vi "catch array get.vi"(11 "main-national data":T1) -> (0 "finish?":bool, 3 "main data out":T1)   [LabVIEW 2019]
uses:
  ctl/main data-national.ctl
  ctl/position set.ctl
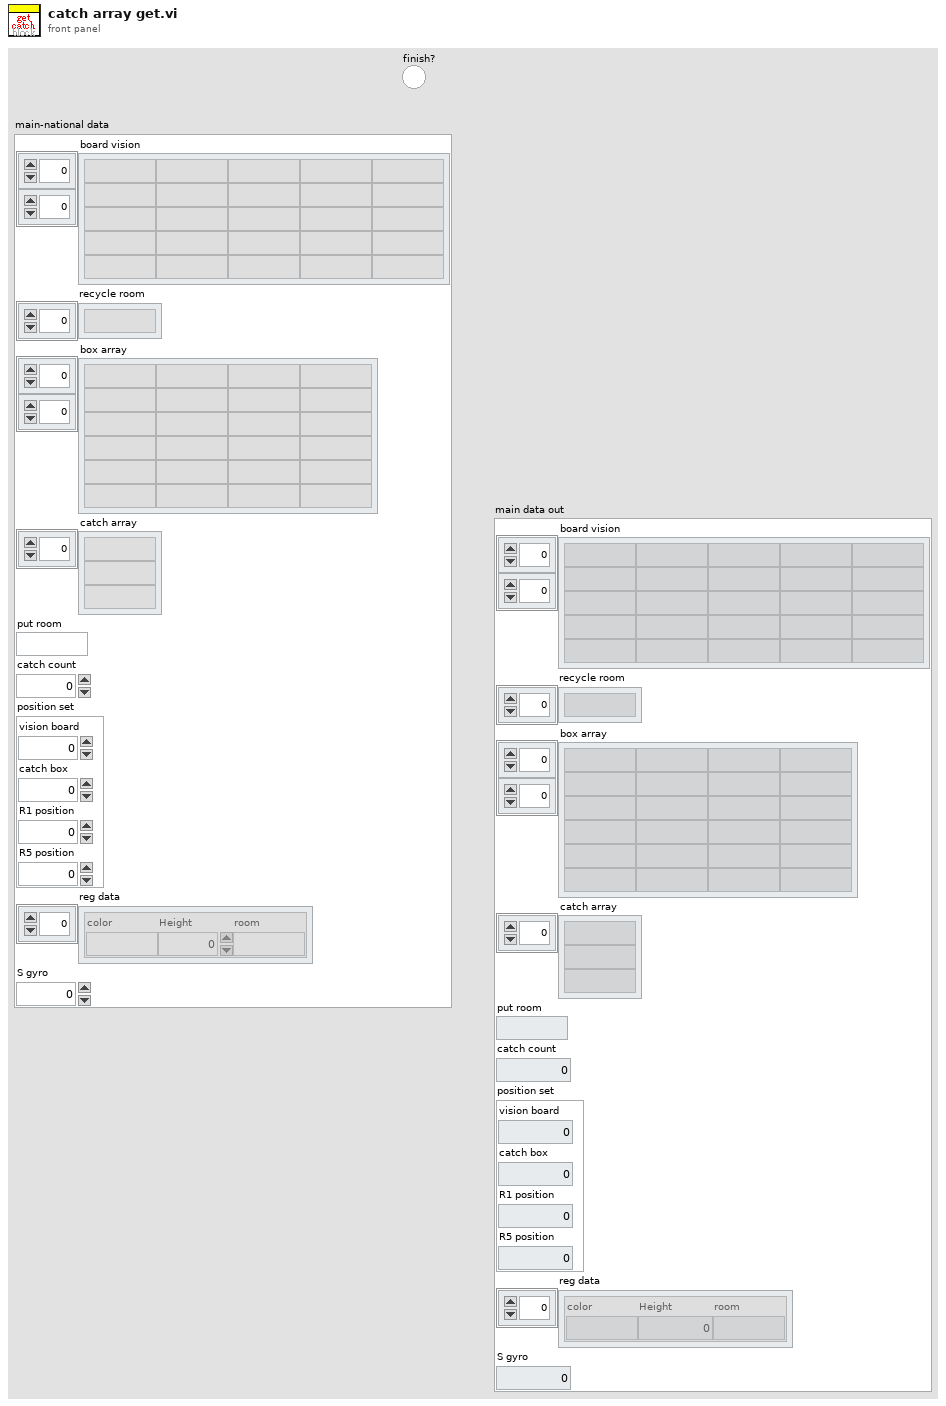
[diagram p1: front panel]
types:
  T1 = typedef "main data-national.ctl" = cluster{"board vision":string[][], "recycle room":string[], "box array":string[][], "catch array":string[], "put room":string, "catch count":dbl, "position set":T2, "reg data":cluster{"color":string, "Height":i32, "room":string}[], "S gyro":dbl}
  T2 = typedef "position set.ctl" = cluster{"vision board":dbl, "catch box":dbl, "R1 position":dbl, "R5 position":dbl}
  T3 = cluster{"color":string, "Height":i32, "room":string}[]
  T4 = cluster{"color":string, "Height":i32, "room":string}
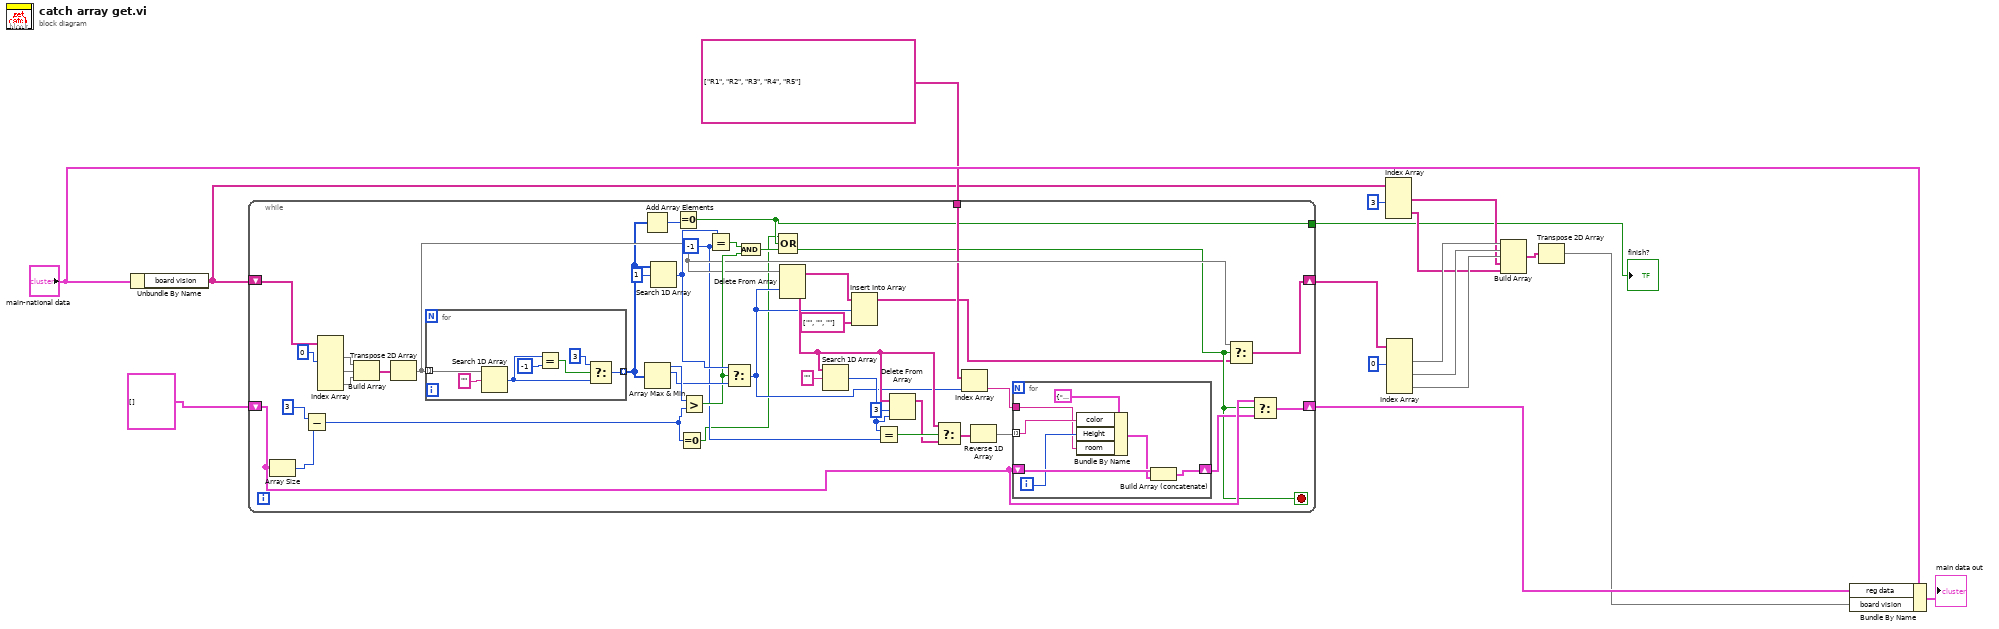
[diagram p0: block diagram]
diagram:
  n1 = Unbundle By Name("main-national data") -> ("board vision"=w10:string[][])
  n2 = while {
    shift-right: [w43] -> w12
    shift-left: w10 -> [w54]
    shift-right: [w31] -> w13
    shift-left: T3 [] ("reg data") -> [w29]
    tunnel: string[] ["R1", "R2", "R3", "R4", "R5"] -> [w33]
    tunnel: [w24] -> w1
    stop <- w25 stop-if-true
    w41 = -1 ("y")
    n3 = Array Size(array=w29) -> (size(s)=w51:i32)
    n4 = Subtract(x=3, y=w51) -> (x-y=w19:i32)
    n5 = Index Array(array=w54, index (col) #1=0 ("disabled index (col)")) -> (element #1=w58:string[], element #2=w56:string[], element #3=w57:string[])  [unwired: 5 in]
    n6 = Build Array(w58, w56, w57) -> (w53:string[][])
    n7 = Transpose 2D Array(2D array=w53) -> (transposed array=w44:string[][])
    n8 = for {
      tunnel: w44 -> [w72] mode=indexing
      tunnel: [w66] -> w27 mode=indexing
      n9 = Search 1D Array(1D array=w72, element="") -> (index of element=w70:i32)  [unwired: 1 in]
      n10 = Equal?(x=w70, y=-1) -> (x = y?=w68:bool)
      n11 = Select(t=3, s=w68, f=w70) -> (s? t:f=w66:i32)
    }
    n12 = Add Array Elements(numeric array=w27) -> (sum=w26:i32)
    n13 = Array Max & Min(array=w27) -> (max value=w50:i32, max index (indices)=w48:i32)  [unwired: 2 out]
    n14 = Search 1D Array(1D array=w27, element=1) -> (index of element=w47:i32)  [unwired: 1 in]
    n15 = Equal To 0?(x=w26) -> (x = 0?=w24:bool)
    n16 = Equal To 0?(x=w19) -> (x = 0?=w18:bool)
    n17 = Greater?(x=w50, y=w19) -> (0:w45:bool)
    n18 = Equal?(x=w47, y=w41) -> (x = y?=w46:bool)
    n19 = Select(t=w47, s=w45, f=w48) -> (s? t:f=w22:i32)
    n20 = And(x=w46, y=w45) -> (x .and. y?=w30:bool)
    n21 = Compound Arithmetic op=OR(w18, w24, w30) -> (w25:bool)
    n22 = Delete From Array(array=w44, index (row)=w22) -> (deleted portion=w39:string[], array with subset deleted=w23:string[][])  [unwired: 2 in]
    n23 = Search 1D Array(1D array=w39, element="") -> (index of element=w37:i32)  [unwired: 1 in]
    n24 = Insert Into Array(array=w23, index (row)=w22, new element=string[] ["", "", ""] ("new element/subarray")) -> (w20:string[][])  [unwired: 1 in]
    n25 = Equal?(x=w37, y=w41) -> (x = y?=w40:bool)
    n26 = Delete From Array(array=w39, length=3, index=w37) -> (array with subset deleted=w36:string[])  [unwired: 1 out]
    n27 = Select(t=w39, s=w40, f=w36) -> (s? t:f=w35:string[])
    n28 = Index Array(array=w33, index=w22) -> (element=w32:string)
    n29 = Reverse 1D Array(array=w35) -> (reversed array=w34:string[])
    n30 = for {
      shift-right: [w64] -> w28
      shift-left: w29 -> [w65]
      tunnel: w34 -> [w62] mode=indexing
      tunnel: w32 -> [w60]
      i -> [w61]
      n31 = Bundle By Name(cluster=T4 {"color"="", "Height"=0, "room"=""} ("Cluster"), "color"=w62, "Height"=w61, "room"=w60) -> (w59:T4)
      n32 = Build Array (concatenate)(w65, w59) -> (w64:T3)
    }
    n33 = Select(t=w44, s=w25, f=w20) -> (s? t:f=w43:string[][])
    n34 = Select(t=w29, s=w25, f=w28) -> (s? t:f=w31:T3)
  }
  "finish?" <- w1
  n35 = Index Array(array=w10, index (col) #1=3 ("disabled index (col)")) -> (element #1=w5:string[], element #2=w4:string[])  [unwired: 3 in]
  n36 = Index Array(array=w12, index (col) #1=0 ("disabled index (col)")) -> (element #1=w8:string[], element #2=w7:string[], element #3=w6:string[])  [unwired: 5 in]
  n37 = Build Array(w8, w7, w6, w5, w4) -> (w3:string[][])
  n38 = Transpose 2D Array(2D array=w3) -> (transposed array=w2:string[][])
  n39 = Bundle By Name(cluster="main-national data", "reg data"=w13, "board vision"=w2) -> (→"main data out":T1)
